vi "Periodic Tasks.vi"(8 "error in":errorcluster) -> ()   [LabVIEW 2016]
doc: "This VI runs in parallel to other tasks. It can contain as many user-defined periodic loops as you need. These can carry out PID or other sorts of timed response."
uses:
  <vilib>/Rock Robotics/WPI/Utilities/WPI_GetSetVariantRefNum.vi
  Robot Global Data.vi
  <vilib>/Rock Robotics/WPI/RobotDrive/WPI_RobotDriveArcadeDrive_Standard(NoSaturation).vi
  <vilib>/Rock Robotics/Network Tables/NT Read Number.vi
  <vilib>/Rock Robotics/Network Tables/NT Write Number.vi
  <vilib>/Rock Robotics/Network Tables/NT Write Numeric Array.vi
  <vilib>/Rock Robotics/Network Tables/NT Write Boolean.vi
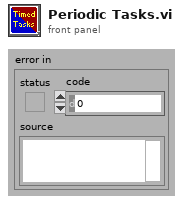
[diagram p1: front panel]
types:
  T1 = enum16{"Init", "Tank Drive", "Left Arcade", "Right Arcade", "Forward", "Vision Alignment", "Climb", "Stop"}
  T2 = enum16{"Init", "wait", "turn left", "turn right", "stop"}
  T3 = typedef "WPI_JoystickDevRef.ctl" = cluster{"Device":T4}
  T4 = typedef "WPI_JoystickDeviceEnum.ctl" = enum16{"USB 0", "USB 1", "USB 2", "USB 3", "USB 4", "USB 5"}
  T5 = cluster{"POVs[0]":i16, "POVs[1]":i16, "POVs[2]":i16, "POVs[3]":i16, "POVs[4]":i16, "POVs[5]":i16, "POVs[6]":i16, "POVs[7]":i16, "POVs[8]":i16}
  T6 = cluster{"Axes[0]":dbl, "Axes[1]":dbl, "Axes[2]":dbl, "Axes[3]":dbl, "Axes[4]":dbl, "Axes[5]":dbl, "Axes[6]":dbl, "Axes[7]":dbl, "Axes[8]":dbl}
  T7 = cluster{"Buttons[0]":bool, "Buttons[1]":bool, "Buttons[2]":bool, "Buttons[3]":bool, "Buttons[4]":bool, "Buttons[5]":bool, "Buttons[6]":bool, "Buttons[7]":bool, "Buttons[8]":bool}
  T8 = typedef "WPI_AccelerometerDevRef.ctl" = cluster{"DevStatus":errorcluster, "Scaling":T9, "Analog Channels":T10, "I2C Bus":T12, "SPI Bus":T13, "Accel Range":T14, "ADXL Axes":T15, "Handle":i32, "Device Address":u8, "Accel Type":enum16{"Analog", "ADXL345 I2C", "ADXL345 SPI", "Internal", "ADXL362 SPI"}}
  T9 = typedef "WPI_AccelerometerScaling.ctl" = cluster{"Gain (VoltsPerG)":dbl, "Center Voltage":dbl}
  T10 = typedef "WPI_AccelerometerAnalogChannels.ctl" = cluster{"X-Axis":T11, "Y-Axis":T11, "Z-Axis":T11}
  T11 = typedef "FPGA_AIChannel.ctl" = enum8{"AI 0", "AI 1", "AI 2", "AI 3", "AI MXP 0", "AI MXP 1", "AI MXP 2", "AI MXP 3", "Invalid"}
  T12 = typedef "i2c_bus.ctl" = enum16{"I2C On-Board", "I2C MXP", "Invalid"}
  T13 = typedef "spi_bus.ctl" = enum16{"SPI On-Board, CS0", "SPI On-Board, CS1", "SPI On-Board, CS2", "SPI On-Board, CS3", "SPI MXP", "Invalid"}
  T14 = typedef "ADXL345 Range.ctl" = u8
  T15 = typedef "WPI_AccelerometerADXL345 Axes.ctl" = cluster{"X-Axis":bool, "Y-Axis":bool, "Z-Axis":bool}
  T16 = typedef "WPI_GyroDevRef.ctl" = cluster{"DevStatus":errorcluster, "Analog Channel":T11, "Offset":dbl, "Gain (VoltsPerDegree/Second)":dbl, "Gyro Type":enum16{"Analog", "XRS450"}, "Handle":i32, "SPI Bus":T13, "Device Found":bool, "Sample Rate":dbl, "Calibrate On Open":bool}
  T17 = cluster{"X-Axis":dbl, "Y-Axis":dbl, "Z-Axis":dbl}
  T18 = typedef "WPI_RobotDriveDevRef.ctl" = cluster{"DevStatus":errorcluster, "Motors[]":T19[], "Square Inputs":bool, "Max Output":dbl}
  T19 = typedef "WPI_MotorControlDeviceRef.ctl" = cluster{"DeviceStatus":errorcluster, "Type":T20, "PWM":cluster{"PWM Channel":T21, "DeadBand":T22}, "CAN":cluster{"Device Number":u8, "SetOutput VI Ref":variant, "GetOutput VI Ref":variant, "Enable VI Ref":variant, "Disable VI Ref":variant, "Data":variant}, "Invert":bool}
  T20 = typedef "WPI_MotorControlType.ctl" = enum16{"PWM", "CAN"}
  T21 = typedef "FPGA_DIOPWMChannel.ctl" = enum8{"PWM 0", "PWM 1", "PWM 2", "PWM 3", "PWM 4", "PWM 5", "PWM 6", "PWM 7", "PWM 8", "PWM 9", "PWM MXP 0", "PWM MXP 1", "PWM MXP 2", "PWM MXP 3", "PWM MXP 4", "PWM MXP 5", "PWM MXP 6", "PWM MXP 7", "PWM MXP 8", "PWM MXP 9", "Invalid"}
  T22 = typedef "WPI_PWMDeadband.ctl" = cluster{"Name":string, "maxPositivePwm":i32, "minPositivePwm":i32, "centerPwm":i32, "maxNegativePwm":i32, "minNegativePwm":i32, "angularRange":u16}
  T23 = enum16{"Init", "Tank Drive", "Left Arcade", "Right Arcade", "Forward", "Back", "Vision Alignment", "Climb", "Stop"}
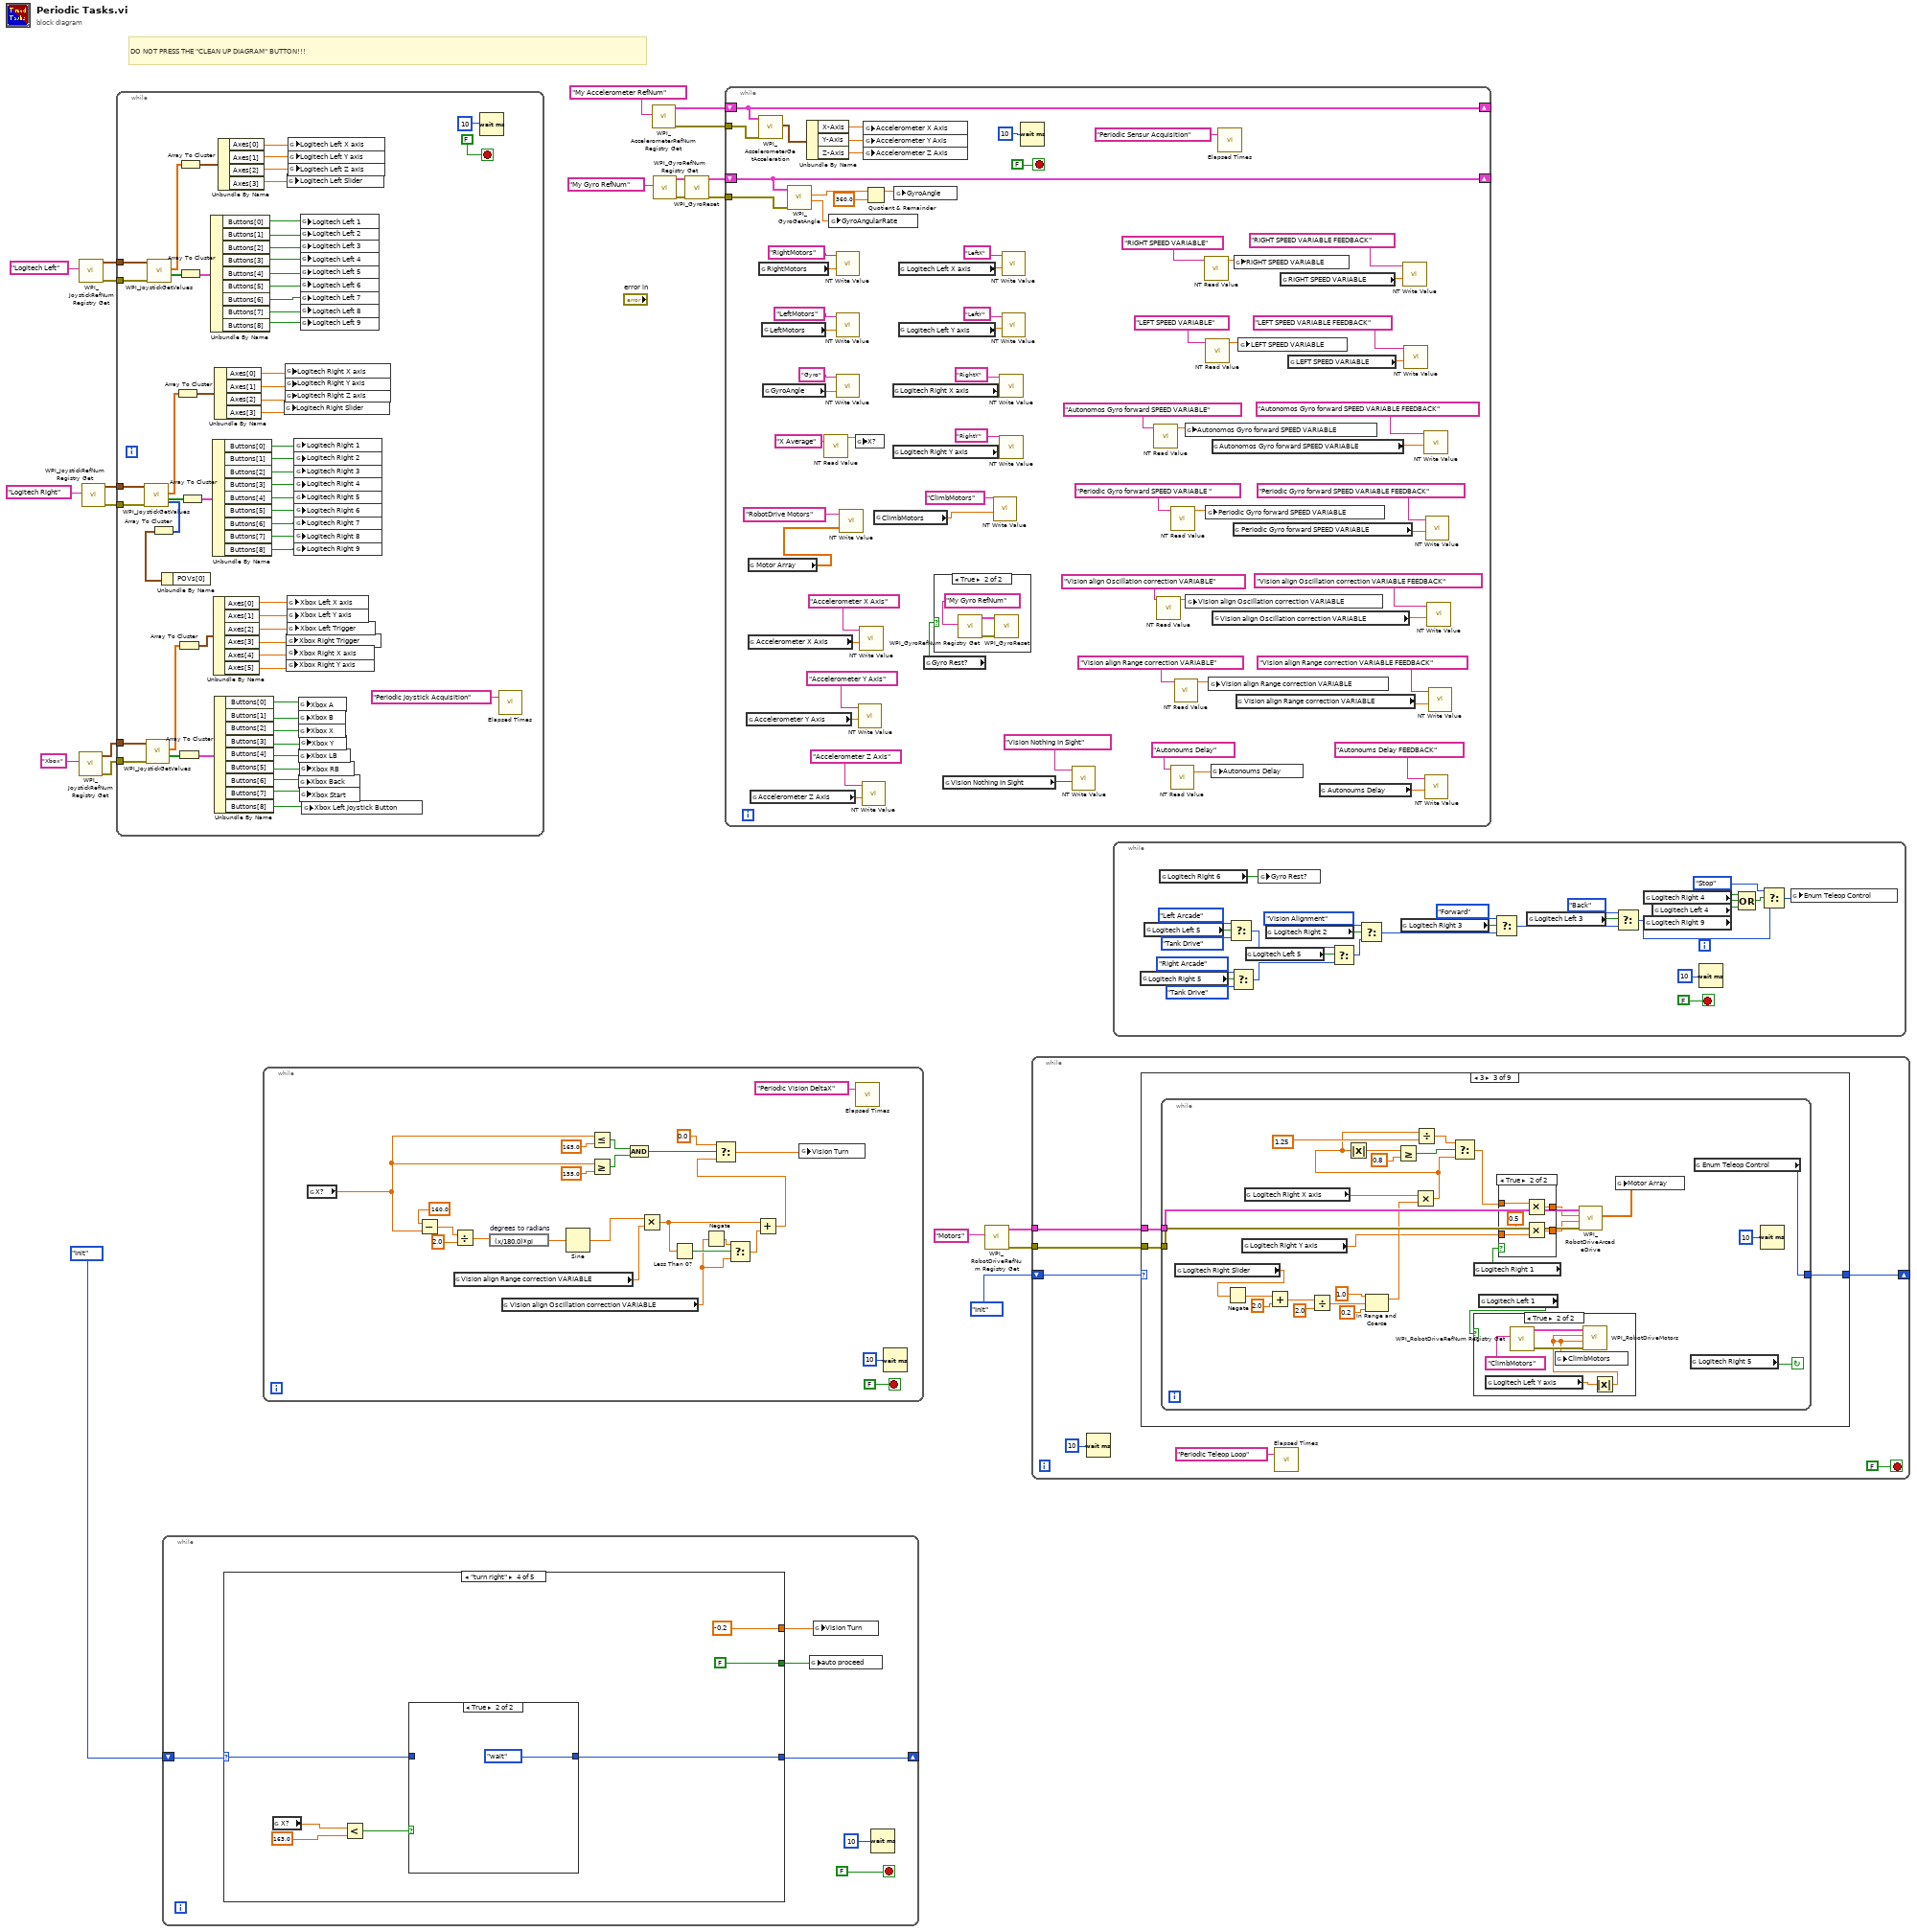
[diagram p0: block diagram]
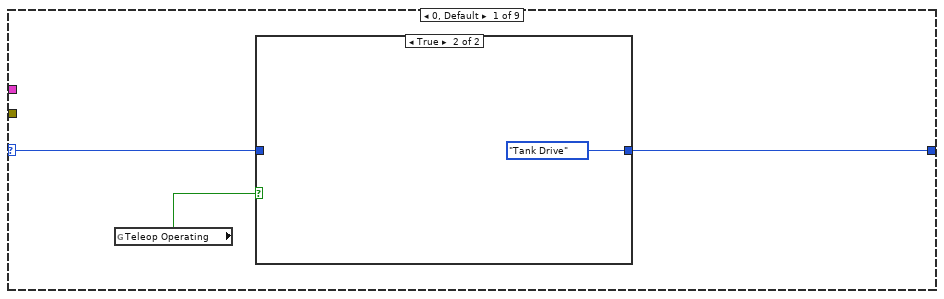
[diagram p2: hidden frame]
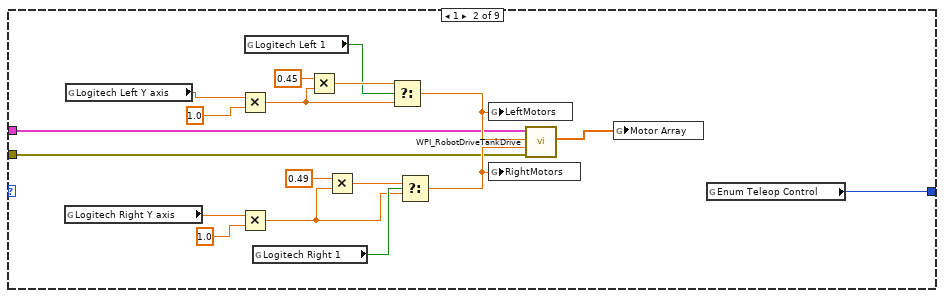
[diagram p4: hidden frame]
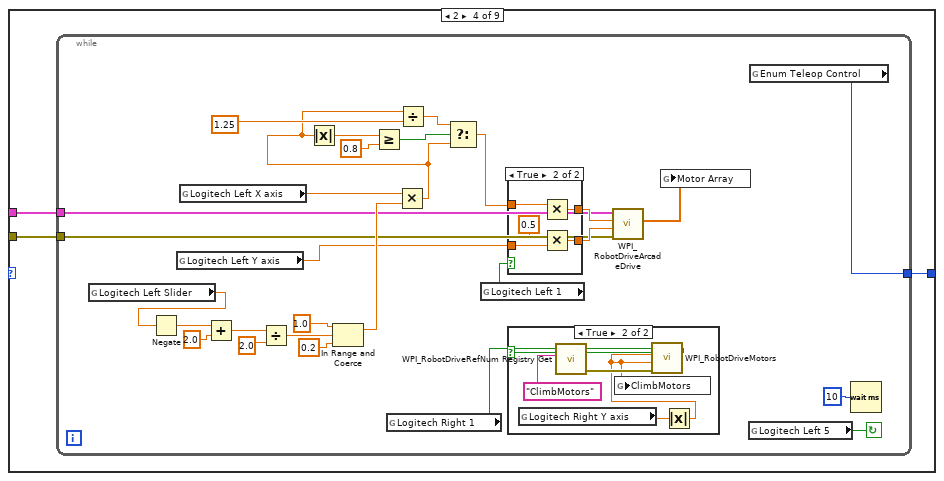
[diagram p7: hidden frame]
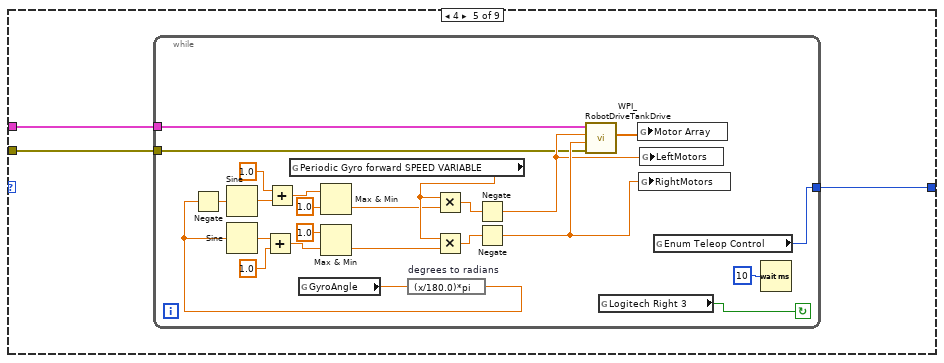
[diagram p10: hidden frame]
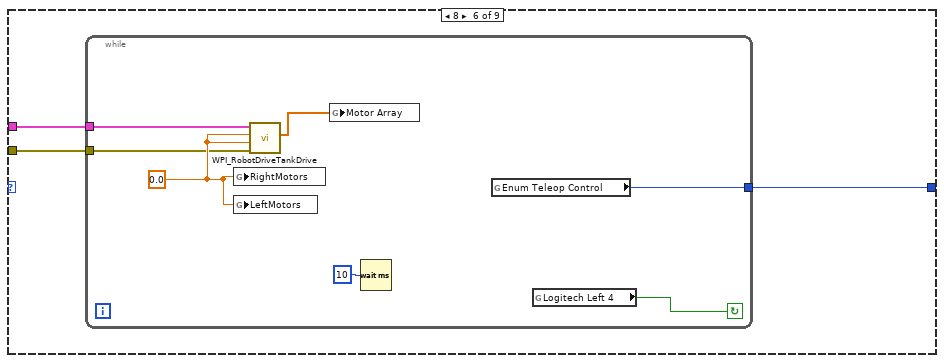
[diagram p11: hidden frame]
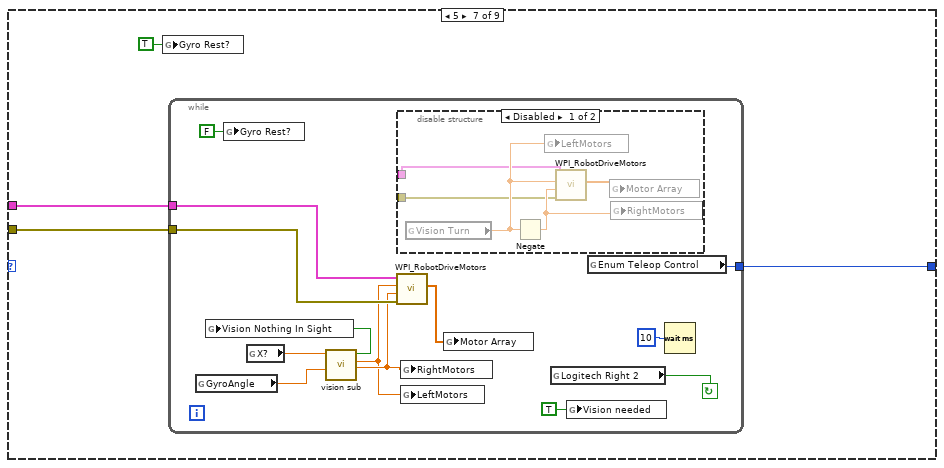
[diagram p12: hidden frame]
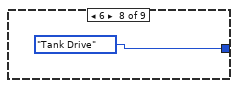
[diagram p14: hidden frame]
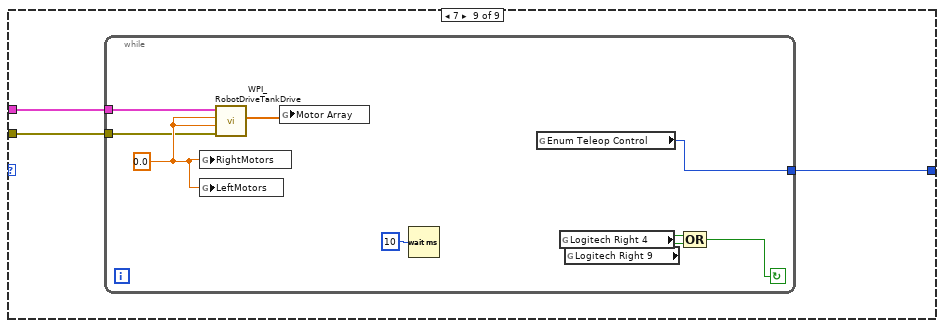
[diagram p15: hidden frame]
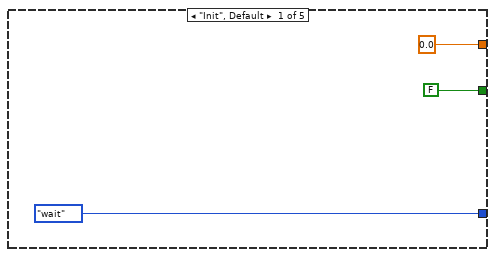
[diagram p16: hidden frame]
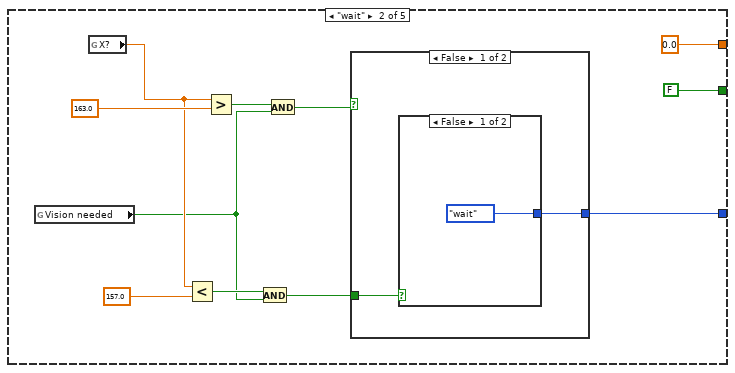
[diagram p17: hidden frame]
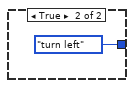
[diagram p18: hidden frame]
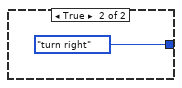
[diagram p19: hidden frame]
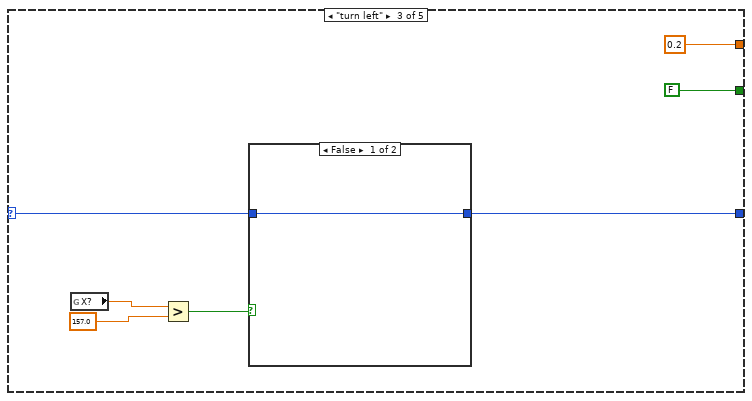
[diagram p20: hidden frame]
diagram:
  # "DO NOT PRESS THE \"CLEAN UP DIAGRAM\" BUTTON!!!"
  n1 = call <vilib>:"WPI_JoystickRefNum Registry Get.vi"("refnum name"="Xbox") -> ("error out"=w15:errorcluster, "JoystickDevRef"=w16:T3)  [unwired: 9 in]
  n2 = call <vilib>:"WPI_JoystickRefNum Registry Get.vi"("refnum name"="Logitech Left") -> ("error out"=w9:errorcluster, "JoystickDevRef"=w10:T3)  [unwired: 9 in]
  n3 = call <vilib>:"WPI_JoystickRefNum Registry Get.vi"("refnum name"="Logitech Right") -> ("error out"=w14:errorcluster, "JoystickDevRef"=w13:T3)  [unwired: 9 in]
  n4 = while {
    tunnel: w16 -> [w77]
    tunnel: w15 -> [w76]
    tunnel: w13 -> [w52]
    tunnel: w14 -> [w53]
    tunnel: w10 -> [w39]
    tunnel: w9 -> [w38]
    stop <- FALSE stop-if-true
    n5 = call <vilib>:"WPI_JoystickGetValues.vi"("error in (no error)"=w53, "JoystickDevRef"=w52) -> ("Buttons"=w64:bool[], "Axes"=w46:dbl[], "POVs"=w26:i16[])  [unwired: 5 in, 2 out]
    n6 = call <vilib>:"WPI_JoystickGetValues.vi"("error in (no error)"=w76, "JoystickDevRef"=w77) -> ("Buttons"=w65:bool[], "Axes"=w84:dbl[])  [unwired: 5 in, 3 out]
    n7 = call <vilib>:"WPI_JoystickGetValues.vi"("error in (no error)"=w38, "JoystickDevRef"=w39) -> ("Buttons"=w27:bool[], "Axes"=w45:dbl[])  [unwired: 5 in, 3 out]
    n8 = Array To Cluster(array=w26) -> (cluster=w25:T5)
    n9 = Unbundle By Name(w25) -> ()  [unwired: 1 out]
    n10 = Array To Cluster(array=w46) -> (cluster=w47:T6)
    n11 = Array To Cluster(array=w84) -> (cluster=w83:T6)
    n12 = Array To Cluster(array=w65) -> (cluster=w75:T7)
    n13 = Array To Cluster(array=w45) -> (cluster=w44:T6)
    n14 = Array To Cluster(array=w27) -> (cluster=w37:T7)
    n15 = Array To Cluster(array=w64) -> (cluster=w54:T7)
    n16 = Unbundle By Name(w37) -> ("Buttons[0]"=w36:bool, "Buttons[1]"=w35:bool, "Buttons[2]"=w34:bool, "Buttons[3]"=w33:bool, "Buttons[4]"=w32:bool, "Buttons[5]"=w31:bool, "Buttons[6]"=w30:bool, "Buttons[7]"=w29:bool, "Buttons[8]"=w28:bool)
    n17 = Unbundle By Name(w54) -> ("Buttons[0]"=w55:bool, "Buttons[1]"=w56:bool, "Buttons[2]"=w57:bool, "Buttons[3]"=w58:bool, "Buttons[4]"=w59:bool, "Buttons[5]"=w60:bool, "Buttons[6]"=w61:bool, "Buttons[7]"=w62:bool, "Buttons[8]"=w63:bool)
    n18 = Unbundle By Name(w83) -> ("Axes[0]"=w24:dbl, "Axes[1]"=w82:dbl, "Axes[2]"=w81:dbl, "Axes[3]"=w80:dbl, "Axes[4]"=w79:dbl, "Axes[5]"=w78:dbl)
    n19 = Unbundle By Name(w75) -> ("Buttons[0]"=w74:bool, "Buttons[1]"=w73:bool, "Buttons[2]"=w72:bool, "Buttons[3]"=w71:bool, "Buttons[4]"=w70:bool, "Buttons[5]"=w69:bool, "Buttons[6]"=w68:bool, "Buttons[7]"=w67:bool, "Buttons[8]"=w66:bool)
    n20 = Unbundle By Name(w47) -> ("Axes[0]"=w48:dbl, "Axes[1]"=w49:dbl, "Axes[2]"=w50:dbl, "Axes[3]"=w51:dbl)
    n21 = Unbundle By Name(w44) -> ("Axes[0]"=w43:dbl, "Axes[1]"=w42:dbl, "Axes[2]"=w41:dbl, "Axes[3]"=w40:dbl)
    n22 = global write "Robot Global Data.vi" "Logitech Right Slider"(w51) -> ()
    n23 = global write "Robot Global Data.vi" "Logitech Right X axis"(w48) -> ()
    n24 = global write "Robot Global Data.vi" "Logitech Right Y axis"(w49) -> ()
    n25 = global write "Robot Global Data.vi" "Logitech Right Z axis"(w50) -> ()
    n26 = global write "Robot Global Data.vi" "Xbox Right Trigger"(w80) -> ()
    n27 = global write "Robot Global Data.vi" "Xbox Right X axis"(w79) -> ()
    n28 = global write "Robot Global Data.vi" "Xbox Right Y axis"(w78) -> ()
    n29 = global write "Robot Global Data.vi" "Logitech Left Slider"(w40) -> ()
    n30 = global write "Robot Global Data.vi" "Xbox Left X axis"(w24) -> ()
    n31 = global write "Robot Global Data.vi" "Xbox Left Y axis"(w82) -> ()
    n32 = global write "Robot Global Data.vi" "Xbox Left Trigger"(w81) -> ()
    n33 = global write "Robot Global Data.vi" "Logitech Left X axis"(w43) -> ()
    n34 = global write "Robot Global Data.vi" "Logitech Left Y axis"(w42) -> ()
    n35 = global write "Robot Global Data.vi" "Logitech Left Z axis"(w41) -> ()
    n36 = global write "Robot Global Data.vi" "Logitech Right 1"(w55) -> ()
    n37 = global write "Robot Global Data.vi" "Logitech Right 2"(w56) -> ()
    n38 = global write "Robot Global Data.vi" "Logitech Right 3"(w57) -> ()
    n39 = global write "Robot Global Data.vi" "Logitech Right 4"(w58) -> ()
    n40 = global write "Robot Global Data.vi" "Logitech Right 5"(w59) -> ()
    n41 = global write "Robot Global Data.vi" "Logitech Right 6"(w60) -> ()
    n42 = global write "Robot Global Data.vi" "Logitech Right 7"(w61) -> ()
    n43 = global write "Robot Global Data.vi" "Logitech Right 8"(w62) -> ()
    n44 = global write "Robot Global Data.vi" "Logitech Right 9"(w63) -> ()
    n45 = global write "Robot Global Data.vi" "Xbox A"(w74) -> ()
    n46 = global write "Robot Global Data.vi" "Xbox B"(w73) -> ()
    n47 = global write "Robot Global Data.vi" "Xbox X"(w72) -> ()
    n48 = global write "Robot Global Data.vi" "Xbox LB"(w70) -> ()
    n49 = global write "Robot Global Data.vi" "Xbox Back"(w68) -> ()
    n50 = global write "Robot Global Data.vi" "Xbox Y"(w71) -> ()
    n51 = global write "Robot Global Data.vi" "Xbox RB"(w69) -> ()
    n52 = global write "Robot Global Data.vi" "Xbox Start"(w67) -> ()
    n53 = global write "Robot Global Data.vi" "Logitech Left 1"(w36) -> ()
    n54 = global write "Robot Global Data.vi" "Logitech Left 2"(w35) -> ()
    n55 = global write "Robot Global Data.vi" "Logitech Left 3"(w34) -> ()
    n56 = global write "Robot Global Data.vi" "Logitech Left 4"(w33) -> ()
    n57 = global write "Robot Global Data.vi" "Logitech Left 5"(w32) -> ()
    n58 = global write "Robot Global Data.vi" "Logitech Left 6"(w31) -> ()
    n59 = global write "Robot Global Data.vi" "Logitech Left 7"(w30) -> ()
    n60 = global write "Robot Global Data.vi" "Logitech Left 8"(w29) -> ()
    n61 = global write "Robot Global Data.vi" "Logitech Left 9"(w28) -> ()
    n62 = global write "Robot Global Data.vi" "Xbox Left Joystick Button"(w66) -> ()
    n63 = Wait (ms)(milliseconds to wait=u32 10) -> ()  [unwired: 1 out]
    n64 = call "Elapsed Times.vi"("Call Name"="Periodic Joystick Acquisition") -> ()  [unwired: 2 in, 1 out]
  }
  n65 = while {
    shift-right: [w89] -> _
    shift-left: T2."Init" -> [w90]
    stop <- FALSE stop-if-true
    n66 = case shown="\"turn right\"" w90 {
      selector: w90 -> [_ _ w115 w124 _]
      tunnel: [T2."wait" w106 w116 w123 w130] -> w89
      tunnel: [FALSE FALSE FALSE FALSE TRUE] -> w88
      tunnel: [0.0 0.0 0.2 -0.2 0.0] -> w87
      frame "Init", Default {
      }
      frame "wait" {
        n67 = global read "Robot Global Data.vi" "Vision needed"() -> (w96:bool)
        n68 = global read "Robot Global Data.vi" "X?"() -> (w101:dbl)
        n69 = Less?(x=w101, y=157.0) -> (x < y?=w99:bool)
        n70 = Greater?(x=w101, y=163.0) -> (0:w100:bool)
        n71 = And(x=w99, y=w96) -> (x .and. y?=w97:bool)
        n72 = And(x=w100, y=w96) -> (x .and. y?=w98:bool)
        n73 = case shown="False" w98 {
          tunnel: [w108 T2."turn right"] -> w106
          tunnel: w97 -> [w107 _]
          frame False {
            n74 = case shown="False" w107 {
              tunnel: [T2."wait" T2."turn left"] -> w108
              frame False {
              }
              frame True {
              }
            }
          }
          frame True {
          }
        }
      }
      frame "turn left" {
        n75 = global read "Robot Global Data.vi" "X?"() -> (w112:dbl)
        n76 = Greater?(x=w112, y=157.0) -> (0:w114:bool)
        n77 = case shown="False" w114 {
          tunnel: [w119 T2."wait"] -> w116
          tunnel: w115 -> [w119 _]
          frame False {
          }
          frame True {
          }
        }
      }
      frame "turn right" {
        n78 = global read "Robot Global Data.vi" "X?"() -> (w125:dbl)
        n79 = Less?(x=w125, y=163.0) -> (x < y?=w127:bool)
        n80 = case shown="True" w127 {
          tunnel: [w128 T2."wait"] -> w123
          tunnel: w124 -> [w128 _]
          frame False {
          }
          frame True {
          }
        }
      }
      frame "stop" {
        n81 = global read "Robot Global Data.vi" "Logitech Right 2"() -> (w131:bool)
        n82 = case shown="False" w131 {
          tunnel: [T2."stop" T2."Init"] -> w130
          frame False {
          }
          frame True {
          }
        }
      }
    }
    n83 = global write "Robot Global Data.vi" "auto proceed"(w88) -> ()
    n84 = global write "Robot Global Data.vi" "Vision Turn"(w87) -> ()
    n85 = Wait (ms)(milliseconds to wait=u32 10) -> ()  [unwired: 1 out]
  }
  n86 = while {
    stop <- FALSE stop-if-true
    n87 = global read "Robot Global Data.vi" "X?"() -> (w155:dbl)
    n88 = Subtract(x=160.0, y=w155) -> (x-y=w151:dbl)
    n89 = Divide(x=w151, y=2.0) -> (x/y=w153:dbl)
    n90 = global read "Robot Global Data.vi" "Vision align Range correction VARIABLE"() -> (w138:dbl)
    n91 = expression code="(x/180.0)*pi" "degrees to radians"(w153) -> (w154:dbl)
    n92 = global read "Robot Global Data.vi" "Vision align Oscillation correction VARIABLE"() -> (w139:dbl)
    n93 = Sine(x=w154) -> (sin(x)=w156:dbl)
    n94 = Less Or Equal?(x=w155, y=165.0) -> (x <= y?=w143:bool)
    n95 = Greater Or Equal?(x=w155, y=155.0) -> (x >= y?=w142:bool)
    n96 = And(x=w143, y=w142) -> (x .and. y?=w145:bool)
    n97 = Multiply(x=w156, y=w138) -> (x*y=w148:dbl)
    n98 = Less Than 0?(x=w148) -> (x < 0?=w146:bool)
    n99 = Negate(x=w139) -> (-x=w149:dbl)
    n100 = Select(t=w149, s=w146, f=w139) -> (s? t:f=w147:dbl)
    n101 = Add(x=w148, y=w147) -> (x+y=w157:dbl)
    n102 = Select(t=0.0, s=w145, f=w157) -> (s? t:f=w137:dbl)
    n103 = global write "Robot Global Data.vi" "Vision Turn"(w137) -> ()
    n104 = call "Elapsed Times.vi"("Call Name"="Periodic Vision DeltaX") -> ()  [unwired: 2 in, 1 out]
    n105 = Wait (ms)(milliseconds to wait=u32 10) -> ()  [unwired: 1 out]
  }
  n106 = call <vilib>:"WPI_AccelerometerRefNum Registry Get.vi"("refnum name"="My Accelerometer RefNum") -> ("error out"=w2:errorcluster, "AccelerometerDevRef"=w3:T8)  [unwired: 9 in]
  n107 = call <vilib>:"WPI_GyroRefNum Registry Get.vi"("refnum name"="My Gyro RefNum") -> ("error out"=w20:errorcluster, "GyroDevRef"=w21:T16)  [unwired: 9 in]
  n108 = call <vilib>:"WPI_GyroReset.vi"("error in"=w20, "GyroDevRef"=w21) -> ("error out"=w18:errorcluster, "GyroDevRef"=w19:T16)  [unwired: 8 in]
  n109 = while {
    shift-right: [w228] -> _
    shift-left: w19 -> [w228]
    tunnel: w18 -> [w227]
    shift-right: [w194] -> _
    shift-left: w3 -> [w194]
    tunnel: w2 -> [w193]
    stop <- FALSE stop-if-true
    n110 = global read "Robot Global Data.vi" "Accelerometer Y Axis"() -> (w165:dbl)
    n111 = global read "Robot Global Data.vi" "Motor Array"() -> (w209:dbl[])
    n112 = global read "Robot Global Data.vi" "Accelerometer X Axis"() -> (w160:dbl)
    n113 = global read "Robot Global Data.vi" "Accelerometer Z Axis"() -> (w162:dbl)
    n114 = call <vilib>:"WPI_AccelerometerGetAcceleration.vi"("error in"=w193, "AccelerometerDevRef"=w194) -> ("Accelerations"=w192:T17)  [unwired: 7 in, 2 out]
    n115 = global read "Robot Global Data.vi" "RightMotors"() -> (w221:dbl)
    n116 = global read "Robot Global Data.vi" "LeftMotors"() -> (w218:dbl)
    n117 = global read "Robot Global Data.vi" "GyroAngle"() -> (w226:dbl)
    n118 = call <vilib>:"WPI_GyroGetAngle.vi"("error in"=w227, "GyroDevRef"=w228) -> ("Angular Rate"=w229:dbl, "Angle"=w208:dbl)  [unwired: 5 in, 3 out]
    n119 = Unbundle By Name(w192) -> ("X-Axis"=w191:dbl, "Y-Axis"=w190:dbl, "Z-Axis"=w189:dbl)
    n120 = call-poly <vilib>:"NT Read Value.vi"("Name"="X Average") -> ("Numeric"=w223:dbl)  [unwired: 9 in, 1 out]
    n121 = global write "Robot Global Data.vi" "GyroAngularRate"(w229) -> ()
    n122 = call-poly <vilib>:"NT Write Value.vi"("Numeric"=w221, "Name"="RightMotors") -> ()  [unwired: 9 in, 1 out]
    n123 = call-poly <vilib>:"NT Write Value.vi"("Numeric"=w218, "Name"="LeftMotors") -> ()  [unwired: 9 in, 1 out]
    n124 = call-poly <vilib>:"NT Write Value.vi"("Numeric"=w226, "Name"="Gyro") -> ()  [unwired: 9 in, 1 out]
    n125 = call-poly <vilib>:"NT Write Value.vi"("Numeric Array"=w209, "Name"="RobotDrive Motors") -> ()  [unwired: 9 in, 1 out]
    n126 = global write "Robot Global Data.vi" "X?"(w223) -> ()
    n127 = call-poly <vilib>:"NT Write Value.vi"("Numeric"=w165, "Name"="Accelerometer Y Axis") -> ()  [unwired: 9 in, 1 out]
    n128 = call-poly <vilib>:"NT Write Value.vi"("Numeric"=w160, "Name"="Accelerometer X Axis") -> ()  [unwired: 9 in, 1 out]
    n129 = call-poly <vilib>:"NT Write Value.vi"("Numeric"=w162, "Name"="Accelerometer Z Axis") -> ()  [unwired: 9 in, 1 out]
    n130 = global write "Robot Global Data.vi" "Accelerometer X Axis"(w191) -> ()
    n131 = global write "Robot Global Data.vi" "Accelerometer Y Axis"(w190) -> ()
    n132 = global write "Robot Global Data.vi" "Accelerometer Z Axis"(w189) -> ()
    n133 = Quotient & Remainder(x=w208, y=360.0) -> (x-y*floor(x/y)=w206:dbl)  [unwired: 1 out]
    n134 = global read "Robot Global Data.vi" "ClimbMotors"() -> (w204:dbl)
    n135 = global read "Robot Global Data.vi" "Logitech Right X axis"() -> (w215:dbl)
    n136 = global read "Robot Global Data.vi" "Logitech Right Y axis"() -> (w216:dbl)
    n137 = global write "Robot Global Data.vi" "GyroAngle"(w206) -> ()
    n138 = global read "Robot Global Data.vi" "Logitech Left X axis"() -> (w220:dbl)
    n139 = global read "Robot Global Data.vi" "Logitech Left Y axis"() -> (w219:dbl)
    n140 = global read "Robot Global Data.vi" "Gyro Rest?"() -> (w203:bool)
    n141 = case shown="True" w203 {
      frame False {
      }
      frame True {
        n142 = call <vilib>:"WPI_GyroRefNum Registry Get.vi"("refnum name"="My Gyro RefNum") -> ("error out"=w234:errorcluster, "GyroDevRef"=w233:T16)  [unwired: 9 in]
        n143 = call <vilib>:"WPI_GyroReset.vi"("error in"=w234, "GyroDevRef"=w233) -> ()  [unwired: 8 in, 2 out]
      }
    }
    n144 = global read "Robot Global Data.vi" "Vision Nothing In Sight"() -> (w166:bool)
    n145 = call-poly <vilib>:"NT Write Value.vi"("Numeric"=w204, "Name"="ClimbMotors") -> ()  [unwired: 9 in, 1 out]
    n146 = call-poly <vilib>:"NT Write Value.vi"("Numeric"=w215, "Name"="RightX") -> ()  [unwired: 9 in, 1 out]
    n147 = call-poly <vilib>:"NT Write Value.vi"("Numeric"=w216, "Name"="RightY") -> ()  [unwired: 9 in, 1 out]
    n148 = call-poly <vilib>:"NT Write Value.vi"("Numeric"=w220, "Name"="LeftX") -> ()  [unwired: 9 in, 1 out]
    n149 = call-poly <vilib>:"NT Write Value.vi"("Numeric"=w219, "Name"="LeftY") -> ()  [unwired: 9 in, 1 out]
    n150 = Wait (ms)(milliseconds to wait=u32 10) -> ()  [unwired: 1 out]
    n151 = call-poly <vilib>:"NT Write Value.vi"("Boolean"=w166, "Name"="Vision Nothing In Sight") -> ()  [unwired: 9 in, 1 out]
    n152 = call-poly <vilib>:"NT Read Value.vi"("Name"="Autonomos Gyro forward SPEED VARIABLE") -> ("Numeric"=w182:dbl)  [unwired: 9 in, 1 out]
    n153 = call-poly <vilib>:"NT Read Value.vi"("Name"="Vision align Oscillation correction VARIABLE") -> ("Numeric"=w180:dbl)  [unwired: 9 in, 1 out]
    n154 = call-poly <vilib>:"NT Read Value.vi"("Name"="Autonoums Delay") -> ("Numeric"=w171:dbl)  [unwired: 9 in, 1 out]
    n155 = call-poly <vilib>:"NT Read Value.vi"("Name"="Periodic Gyro forward SPEED VARIABLE ") -> ("Numeric"=w186:dbl)  [unwired: 9 in, 1 out]
    n156 = call-poly <vilib>:"NT Read Value.vi"("Name"="Vision align Range correction VARIABLE") -> ("Numeric"=w176:dbl)  [unwired: 9 in, 1 out]
    n157 = global write "Robot Global Data.vi" "Autonomos Gyro forward SPEED VARIABLE"(w182) -> ()
    n158 = global write "Robot Global Data.vi" "Vision align Oscillation correction VARIABLE"(w180) -> ()
    n159 = call-poly <vilib>:"NT Read Value.vi"("Name"="RIGHT SPEED VARIABLE") -> ("Numeric"=w201:dbl)  [unwired: 9 in, 1 out]
    n160 = call-poly <vilib>:"NT Read Value.vi"("Name"="LEFT SPEED VARIABLE") -> ("Numeric"=w197:dbl)  [unwired: 9 in, 1 out]
    n161 = global write "Robot Global Data.vi" "Periodic Gyro forward SPEED VARIABLE"(w186) -> ()
    n162 = global write "Robot Global Data.vi" "Vision align Range correction VARIABLE"(w176) -> ()
    n163 = global write "Robot Global Data.vi" "Autonoums Delay"(w171) -> ()
    n164 = global read "Robot Global Data.vi" "Autonomos Gyro forward SPEED VARIABLE"() -> (w184:dbl)
    n165 = global read "Robot Global Data.vi" "Vision align Oscillation correction VARIABLE"() -> (w178:dbl)
    n166 = call "Elapsed Times.vi"("Call Name"="Periodic Sensur Acquisition") -> ()  [unwired: 2 in, 1 out]
    n167 = global read "Robot Global Data.vi" "Periodic Gyro forward SPEED VARIABLE"() -> (w185:dbl)
    n168 = global write "Robot Global Data.vi" "RIGHT SPEED VARIABLE"(w201) -> ()
    n169 = global read "Robot Global Data.vi" "Vision align Range correction VARIABLE"() -> (w177:dbl)
    n170 = global write "Robot Global Data.vi" "LEFT SPEED VARIABLE"(w197) -> ()
    n171 = global read "Robot Global Data.vi" "RIGHT SPEED VARIABLE"() -> (w199:dbl)
    n172 = global read "Robot Global Data.vi" "LEFT SPEED VARIABLE"() -> (w198:dbl)
    n173 = global read "Robot Global Data.vi" "Autonoums Delay"() -> (w170:dbl)
    n174 = call-poly <vilib>:"NT Write Value.vi"("Numeric"=w199, "Name"="RIGHT SPEED VARIABLE FEEDBACK") -> ()  [unwired: 9 in, 1 out]
    n175 = call-poly <vilib>:"NT Write Value.vi"("Numeric"=w198, "Name"="LEFT SPEED VARIABLE FEEDBACK") -> ()  [unwired: 9 in, 1 out]
    n176 = call-poly <vilib>:"NT Write Value.vi"("Numeric"=w184, "Name"="Autonomos Gyro forward SPEED VARIABLE FEEDBACK") -> ()  [unwired: 9 in, 1 out]
    n177 = call-poly <vilib>:"NT Write Value.vi"("Numeric"=w170, "Name"="Autonoums Delay FEEDBACK") -> ()  [unwired: 9 in, 1 out]
    n178 = call-poly <vilib>:"NT Write Value.vi"("Numeric"=w185, "Name"="Periodic Gyro forward SPEED VARIABLE FEEDBACK") -> ()  [unwired: 9 in, 1 out]
    n179 = call-poly <vilib>:"NT Write Value.vi"("Numeric"=w178, "Name"="Vision align Oscillation correction VARIABLE FEEDBACK") -> ()  [unwired: 9 in, 1 out]
    n180 = call-poly <vilib>:"NT Write Value.vi"("Numeric"=w177, "Name"="Vision align Range correction VARIABLE FEEDBACK") -> ()  [unwired: 9 in, 1 out]
  }
  n181 = call <vilib>:"WPI_RobotDriveRefNum Registry Get.vi"("refnum name"="Motors") -> ("error out"=w5:errorcluster, "RobotDriveDevRef"=w6:T18)  [unwired: 9 in]
  n182 = while {
    tunnel: w6 -> [w241]
    tunnel: w5 -> [w240]
    shift-right: [w236] -> _
    shift-left: T1."Init" -> [w237]
    stop <- FALSE stop-if-true
    n183 = Wait (ms)(milliseconds to wait=u32 10) -> ()  [unwired: 1 out]
    n184 = case shown="3" w237 {
      selector: w237 -> [w242 _ _ _ _ _ _ _ _]
      tunnel: w241 -> [_ w249 w267 w310 w352 w380 w391 _ w413]
      tunnel: w240 -> [_ w248 w266 w309 w353 w379 w390 _ w412]
      tunnel: [w243 w247 w265 w308 w351 w378 w389 T1."Tank Drive" w411] -> w236
      frame 0, Default {
        n185 = global read "Robot Global Data.vi" "Teleop Operating"() -> (w244:bool)
        n186 = case shown="True" w244 {
          tunnel: [w245 T1."Tank Drive"] -> w243
          tunnel: w242 -> [w245 _]
          frame False {
          }
          frame True {
          }
        }
      }
      frame 1 {
        n187 = global read "Robot Global Data.vi" "Logitech Right Y axis"() -> (w261:dbl)
        n188 = global read "Robot Global Data.vi" "Logitech Left Y axis"() -> (w264:dbl)
        n189 = Multiply(x=w264, y=1.0) -> (x*y=w258:dbl)
        n190 = Multiply(x=w261, y=1.0) -> (x*y=w254:dbl)
        n191 = global read "Robot Global Data.vi" "Logitech Left 1"() -> (w253:bool)
        n192 = global read "Robot Global Data.vi" "Logitech Right 1"() -> (w255:bool)
        n193 = Multiply(x=0.45 ("y"), y=w258) -> (x*y=w259:dbl)
        n194 = Multiply(x=0.49 ("y"), y=w254) -> (x*y=w257:dbl)
        n195 = Select(t=w259, s=w253, f=w258) -> (s? t:f=w252:dbl)
        n196 = Select(t=w257, s=w255, f=w254) -> (s? t:f=w251:dbl)
        n197 = global write "Robot Global Data.vi" "LeftMotors"(w252) -> ()
        n198 = global write "Robot Global Data.vi" "RightMotors"(w251) -> ()
        n199 = call <vilib>:"WPI_RobotDriveTankDrive.vi"("error in (no error)"=w248, "Right axis value"=w251, "Left axis value"=w252, "RobotDriveDevRef"=w249) -> ("Motor Values"=w250:dbl[])  [unwired: 5 in, 2 out]
        n200 = global write "Robot Global Data.vi" "Motor Array"(w250) -> ()
        n201 = global read "Robot Global Data.vi" "Enum Teleop Control"() -> (w247:u16)
      }
      frame 3 {
        n202 = while {
          tunnel: w267 -> [w294]
          tunnel: w266 -> [w293]
          tunnel: [w290] -> w265
          stop <- w292 continue-if-true
          n203 = global read "Robot Global Data.vi" "Logitech Right Slider"() -> (w282:dbl)
          n204 = Negate(x=w282) -> (-x=w286:dbl)
          n205 = global read "Robot Global Data.vi" "Logitech Right Y axis"() -> (w277:dbl)
          n206 = global read "Robot Global Data.vi" "Logitech Right X axis"() -> (w281:dbl)
          n207 = Add(x=w286, y=2.0) -> (x+y=w287:dbl)
          n208 = Divide(x=w287, y=2.0) -> (x/y=w284:dbl)
          n209 = In Range and Coerce(upper limit=1.0, x=w284, lower limit=0.2) -> (coerced(x)=w283:dbl)  [unwired: 1 out]
          n210 = Multiply(x=w281, y=w283) -> (x*y=w273:dbl)
          n211 = Absolute Value(x=w273) -> (abs(x)=w272:dbl)
          n212 = Greater Or Equal?(x=w272, y=0.8) -> (x >= y?=w276:bool)
          n213 = Divide(x=w273, y=1.25) -> (x/y=w275:dbl)
          n214 = Select(t=w275, s=w276, f=w273) -> (s? t:f=w271:dbl)
          n215 = global read "Robot Global Data.vi" "Logitech Right 1"() -> (w268:bool)
          n216 = global read "Robot Global Data.vi" "Logitech Left 1"() -> (w289:bool)
          n217 = case shown="True" w289 {
            frame False {
            }
            frame True {
              n218 = global read "Robot Global Data.vi" "Logitech Left Y axis"() -> (w305:dbl)
              n219 = call <vilib>:"WPI_RobotDriveRefNum Registry Get.vi"("refnum name"="ClimbMotors") -> ("error out"=w306:errorcluster, "RobotDriveDevRef"=w307:T18)  [unwired: 9 in]
              n220 = Absolute Value(x=w305) -> (abs(x)=w304:dbl)
              n221 = global write "Robot Global Data.vi" "ClimbMotors"(w304) -> ()
              n222 = call <vilib>:"WPI_RobotDriveMotors.vi"("error in (no error)"=w306, "RightSpeed"=w304, "LeftSpeed"=w304, "RobotDriveDevRef"=w307) -> ()  [unwired: 8 out]
            }
          }
          n223 = case shown="True" w268 {
            tunnel: w271 -> [w297 w301]
            tunnel: w277 -> [w296 w300]
            tunnel: [w296 w299] -> w270
            tunnel: [w297 w298] -> w269
            frame False {
            }
            frame True {
              w302 = 0.5 ("y")
              n224 = Multiply(x=w301, y=w302) -> (x*y=w298:dbl)
              n225 = Multiply(x=w302, y=w300) -> (x*y=w299:dbl)
            }
          }
          n226 = call-poly <vilib>:"WPI_RobotDriveArcadeDrive.vi"("error in (no error)"=w293, "Y axis value"=w270, "X axis value"=w269, "RobotDriveDevRef"=w294) -> ("Motor Values"=w295:dbl[])  [unwired: 5 in, 2 out]
          n227 = global write "Robot Global Data.vi" "Motor Array"(w295) -> ()
          n228 = global read "Robot Global Data.vi" "Logitech Right 5"() -> (w292:bool)
          n229 = global read "Robot Global Data.vi" "Enum Teleop Control"() -> (w290:u16)
          n230 = Wait (ms)(milliseconds to wait=u32 10) -> ()  [unwired: 1 out]
        }
      }
      frame 2 {
        n231 = while {
          tunnel: w310 -> [w311]
          tunnel: w309 -> [w312]
          tunnel: [w336] -> w308
          stop <- w338 continue-if-true
          n232 = global read "Robot Global Data.vi" "Logitech Left Slider"() -> (w327:dbl)
          n233 = Negate(x=w327) -> (-x=w331:dbl)
          n234 = global read "Robot Global Data.vi" "Logitech Left Y axis"() -> (w322:dbl)
          n235 = global read "Robot Global Data.vi" "Logitech Left X axis"() -> (w326:dbl)
          n236 = Add(x=w331, y=2.0) -> (x+y=w332:dbl)
          n237 = Divide(x=w332, y=2.0) -> (x/y=w329:dbl)
          n238 = In Range and Coerce(upper limit=1.0, x=w329, lower limit=0.2) -> (coerced(x)=w328:dbl)  [unwired: 1 out]
          n239 = global read "Robot Global Data.vi" "Logitech Right 1"() -> (w334:bool)
          n240 = Multiply(x=w326, y=w328) -> (x*y=w318:dbl)
          n241 = Absolute Value(x=w318) -> (abs(x)=w317:dbl)
          n242 = Greater Or Equal?(x=w317, y=0.8) -> (x >= y?=w321:bool)
          n243 = Divide(x=w318, y=1.25) -> (x/y=w320:dbl)
          n244 = Select(t=w320, s=w321, f=w318) -> (s? t:f=w316:dbl)
          n245 = global read "Robot Global Data.vi" "Logitech Left 1"() -> (w313:bool)
          n246 = case shown="True" w313 {
            tunnel: w316 -> [w340 w344]
            tunnel: w322 -> [w339 w343]
            tunnel: [w339 w342] -> w315
            tunnel: [w340 w341] -> w314
            frame False {
            }
            frame True {
              w345 = 0.5 ("y")
              n247 = Multiply(x=w344, y=w345) -> (x*y=w341:dbl)
              n248 = Multiply(x=w345, y=w343) -> (x*y=w342:dbl)
            }
          }
          n249 = case shown="True" w334 {
            frame False {
            }
            frame True {
              n250 = global read "Robot Global Data.vi" "Logitech Right Y axis"() -> (w348:dbl)
              n251 = call <vilib>:"WPI_RobotDriveRefNum Registry Get.vi"("refnum name"="ClimbMotors") -> ("error out"=w349:errorcluster, "RobotDriveDevRef"=w350:T18)  [unwired: 9 in]
              n252 = Absolute Value(x=w348) -> (abs(x)=w347:dbl)
              n253 = global write "Robot Global Data.vi" "ClimbMotors"(w347) -> ()
              n254 = call <vilib>:"WPI_RobotDriveMotors.vi"("error in (no error)"=w349, "RightSpeed"=w347, "LeftSpeed"=w347, "RobotDriveDevRef"=w350) -> ()  [unwired: 8 out]
            }
          }
          n255 = call-poly <vilib>:"WPI_RobotDriveArcadeDrive.vi"("error in (no error)"=w312, "Y axis value"=w315, "X axis value"=w314, "RobotDriveDevRef"=w311) -> ("Motor Values"=w335:dbl[])  [unwired: 5 in, 2 out]
          n256 = global write "Robot Global Data.vi" "Motor Array"(w335) -> ()
          n257 = global read "Robot Global Data.vi" "Logitech Left 5"() -> (w338:bool)
          n258 = global read "Robot Global Data.vi" "Enum Teleop Control"() -> (w336:u16)
          n259 = Wait (ms)(milliseconds to wait=u32 10) -> ()  [unwired: 1 out]
        }
      }
      frame 4 {
        n260 = while {
          tunnel: w353 -> [w355]
          tunnel: w352 -> [w356]
          tunnel: [w354] -> w351
          stop <- w377 continue-if-true
          n261 = global read "Robot Global Data.vi" "Periodic Gyro forward SPEED VARIABLE"() -> (w375:dbl)
          n262 = global read "Robot Global Data.vi" "GyroAngle"() -> (w365:dbl)
          n263 = expression code="(x/180.0)*pi" "degrees to radians"(w365) -> (w366:dbl)
          n264 = Negate(x=w366) -> (-x=w360:dbl)
          n265 = Sine(x=w360) -> (sin(x)=w371:dbl)
          n266 = Sine(x=w366) -> (sin(x)=w369:dbl)
          n267 = Add(x=w369, y=1.0 ("x")) -> (x+y=w370:dbl)
          n268 = Add(x=1.0, y=w371) -> (x+y=w372:dbl)
          n269 = Max & Min(x=w372, y=1.0) -> (min(x,y)=w362:dbl)  [unwired: 1 out]
          n270 = Max & Min(x=1.0, y=w370) -> (min(x,y)=w361:dbl)  [unwired: 1 out]
          n271 = Multiply(x=w375, y=w362) -> (x*y=w363:dbl)
          n272 = Multiply(x=w375, y=w361) -> (x*y=w364:dbl)
          n273 = Negate(x=w363) -> (-x=w373:dbl)
          n274 = Negate(x=w364) -> (-x=w374:dbl)
          n275 = call <vilib>:"WPI_RobotDriveTankDrive.vi"("error in (no error)"=w355, "Right axis value"=w374, "Left axis value"=w373, "RobotDriveDevRef"=w356) -> ("Motor Values"=w357:dbl[])  [unwired: 5 in, 2 out]
          n276 = global read "Robot Global Data.vi" "Logitech Right 3"() -> (w377:bool)
          n277 = global write "Robot Global Data.vi" "Motor Array"(w357) -> ()
          n278 = global write "Robot Global Data.vi" "RightMotors"(w374) -> ()
          n279 = global write "Robot Global Data.vi" "LeftMotors"(w373) -> ()
          n280 = global read "Robot Global Data.vi" "Enum Teleop Control"() -> (w354:u16)
          n281 = Wait (ms)(milliseconds to wait=u32 10) -> ()  [unwired: 1 out]
        }
      }
      frame 8 {
        n282 = while {
          tunnel: w379 -> [w385]
          tunnel: w380 -> [w384]
          tunnel: [w383] -> w378
          stop <- w381 continue-if-true
          w386 = 0.0 ("Right axis value")
          n283 = global write "Robot Global Data.vi" "RightMotors"(w386) -> ()
          n284 = global write "Robot Global Data.vi" "LeftMotors"(w386) -> ()
          n285 = call <vilib>:"WPI_RobotDriveTankDrive.vi"("error in (no error)"=w385, "Right axis value"=w386, "Left axis value"=w386, "RobotDriveDevRef"=w384) -> ("Motor Values"=w387:dbl[])  [unwired: 5 in, 2 out]
          n286 = global write "Robot Global Data.vi" "Motor Array"(w387) -> ()
          n287 = Wait (ms)(milliseconds to wait=u32 10) -> ()  [unwired: 1 out]
          n288 = global read "Robot Global Data.vi" "Enum Teleop Control"() -> (w383:u16)
          n289 = global read "Robot Global Data.vi" "Logitech Left 4"() -> (w381:bool)
        }
      }
      frame 5 {
        n290 = global write "Robot Global Data.vi" "Gyro Rest?"(TRUE ("Gyro Rest?")) -> ()
        n291 = while {
          tunnel: w391 -> [w397]
          tunnel: w390 -> [w396]
          tunnel: [w404] -> w389
          stop <- w403 continue-if-true
          n292 = global read "Robot Global Data.vi" "GyroAngle"() -> (w400:dbl)
          n293 = global write "Robot Global Data.vi" "Gyro Rest?"(FALSE ("Gyro Rest?")) -> ()
          n294 = global read "Robot Global Data.vi" "X?"() -> (w399:dbl)
          n295 = call "vision sub.vi"("Gyro Angle"=w400, "X? Input"=w399) -> ("Right Motors"=w394:dbl, "Left Motors"=w393:dbl, "Nothing In Sight"=w395:bool)  [unwired: 7 in]
          n296 = global write "Robot Global Data.vi" "Vision Nothing In Sight"(w395) -> ()
          n297 = call <vilib>:"WPI_RobotDriveMotors.vi"("error in (no error)"=w396, "RightSpeed"=w394, "LeftSpeed"=w393, "RobotDriveDevRef"=w397) -> ("Motor Values"=w398:dbl[])  [unwired: 7 out]
          n298 = disable-structure shown="Disabled" {
            disable-tunnel: _ -> [w406 _]
            disable-tunnel: _ -> [w405 _]
            frame Disabled {
              n299 = global read "Robot Global Data.vi" "Vision Turn"() -> (w408:dbl)
              n300 = Negate(x=w408) -> (-x=w407:dbl)
              n301 = global write "Robot Global Data.vi" "LeftMotors"(w408) -> ()
              n302 = call <vilib>:"WPI_RobotDriveMotors.vi"("error in (no error)"=w405, "RightSpeed"=w407, "LeftSpeed"=w408, "RobotDriveDevRef"=w406) -> ("Motor Values"=w409:dbl[])  [unwired: 7 out]
              n303 = global write "Robot Global Data.vi" "Motor Array"(w409) -> ()
              n304 = global write "Robot Global Data.vi" "RightMotors"(w407) -> ()
            }
            frame Enabled {
            }
          }
          n305 = global write "Robot Global Data.vi" "RightMotors"(w394) -> ()
          n306 = global write "Robot Global Data.vi" "LeftMotors"(w393) -> ()
          n307 = global write "Robot Global Data.vi" "Motor Array"(w398) -> ()
          n308 = global read "Robot Global Data.vi" "Logitech Right 2"() -> (w403:bool)
          n309 = global write "Robot Global Data.vi" "Vision needed"(TRUE ("Vision needed")) -> ()
          n310 = global read "Robot Global Data.vi" "Enum Teleop Control"() -> (w404:u16)
          n311 = Wait (ms)(milliseconds to wait=u32 10) -> ()  [unwired: 1 out]
        }
      }
      frame 6 {
      }
      frame 7 {
        n312 = while {
          tunnel: w413 -> [w420]
          tunnel: w412 -> [w419]
          tunnel: [w415] -> w411
          stop <- w416 continue-if-true
          w421 = 0.0 ("Right axis value")
          n313 = global write "Robot Global Data.vi" "RightMotors"(w421) -> ()
          n314 = global write "Robot Global Data.vi" "LeftMotors"(w421) -> ()
          n315 = call <vilib>:"WPI_RobotDriveTankDrive.vi"("error in (no error)"=w419, "Right axis value"=w421, "Left axis value"=w421, "RobotDriveDevRef"=w420) -> ("Motor Values"=w422:dbl[])  [unwired: 5 in, 2 out]
          n316 = global write "Robot Global Data.vi" "Motor Array"(w422) -> ()
          n317 = Wait (ms)(milliseconds to wait=u32 10) -> ()  [unwired: 1 out]
          n318 = global read "Robot Global Data.vi" "Enum Teleop Control"() -> (w415:u16)
          n319 = global read "Robot Global Data.vi" "Logitech Right 4"() -> (w417:bool)
          n320 = global read "Robot Global Data.vi" "Logitech Right 9"() -> (w418:bool)
          n321 = Compound Arithmetic op=OR(w417, w418) -> (w416:bool)
        }
      }
    }
    n322 = call "Elapsed Times.vi"("Call Name"="Periodic Teleop Loop") -> ()  [unwired: 2 in, 1 out]
  }
  n323 = while {
    stop <- FALSE stop-if-true
    n324 = global read "Robot Global Data.vi" "Logitech Right 5"() -> (w441:bool)
    n325 = global read "Robot Global Data.vi" "Logitech Left 5"() -> (w440:bool)
    n326 = global read "Robot Global Data.vi" "Logitech Right 6"() -> (w423:bool)
    n327 = Select(t=T1."Left Arcade", s=w440, f=T1."Tank Drive") -> (s? t:f=w431:T1)
    n328 = Select(t=T1."Right Arcade", s=w441, f=T1."Tank Drive") -> (s? t:f=w430:T1)
    n329 = global read "Robot Global Data.vi" "Logitech Left 5"() -> (w442:bool)
    n330 = global write "Robot Global Data.vi" "Gyro Rest?"(w423) -> ()
    n331 = global read "Robot Global Data.vi" "Logitech Right 2"() -> (w443:bool)
    n332 = Select(t=w431, s=w442, f=w430) -> (s? t:f=w438:T1)
    n333 = Select(t=T1."Vision Alignment", s=w443, f=w438) -> (s? t:f=w439:T1)
    n334 = global read "Robot Global Data.vi" "Logitech Right 3"() -> (w444:bool)
    n335 = Select(t=T1."Forward", s=w444, f=w439) -> (s? t:f=w426:T1)
    n336 = global read "Robot Global Data.vi" "Logitech Left 3"() -> (w427:bool)
    n337 = Select(t=T23."Back", s=w427, f=w426) -> (s? t:f=w425:u16)
    n338 = global read "Robot Global Data.vi" "Logitech Right 4"() -> (w445:bool)
    n339 = global read "Robot Global Data.vi" "Logitech Right 9"() -> (w424:bool)
    n340 = global read "Robot Global Data.vi" "Logitech Left 4"() -> (w446:bool)
    n341 = Wait (ms)(milliseconds to wait=u32 10) -> ()  [unwired: 1 out]
    n342 = Compound Arithmetic op=OR(w445, w446, w424) -> (w447:bool)
    n343 = Select(t=T1."Stop", s=w447, f=w425) -> (s? t:f=w448:u16)
    n344 = global write "Robot Global Data.vi" "Enum Teleop Control"(w448) -> ()
  }
